vi "GetCalibration.vi"(8 "error in (no error)":errorcluster, 11 "ByteGSWebAPI-V0 in":refnum<class "ByteGSWebAPI-V0.lvclass">) -> (0 "error out":errorcluster, 3 "ByteGSWebAPI-V0 out":refnum<class "ByteGSWebAPI-V0.lvclass">, 4 "body":string, 6 "headers":string)   [LabVIEW 2019, in "ByteGSWebAPI.lvlib" / "ByteGSWebAPI-V0.lvclass"]
uses:
  ByteGSWebAPI-V0.lvclass
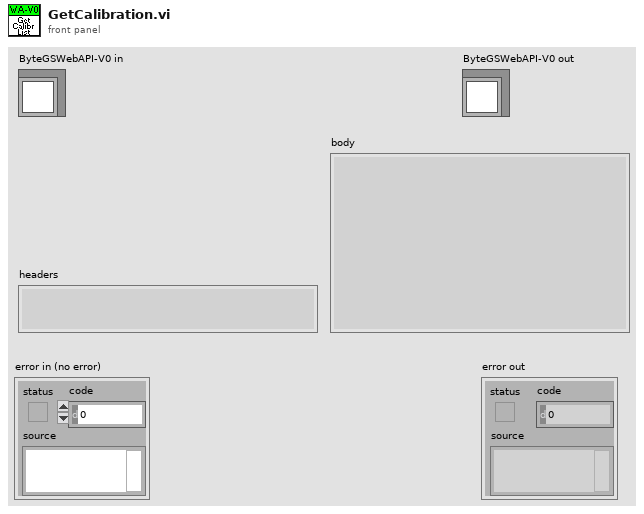
[diagram p1: front panel]
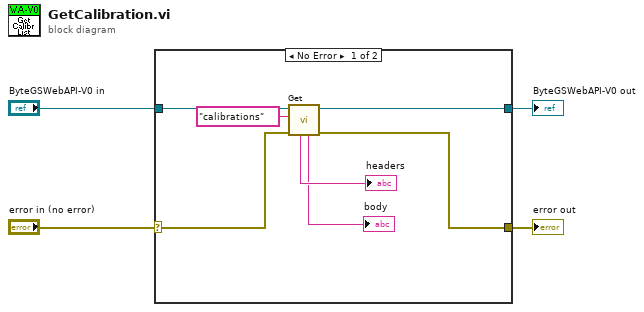
[diagram p0: block diagram]
diagram:
  n1 = case shown="No Error" "error in (no error)" {
    selector: "error in (no error)" -> [w8 w13]
    tunnel: [w5 w13] -> w3
    tunnel: [w10 w12] -> w1
    tunnel: "ByteGSWebAPI-V0 in" -> [w11 w12]
    frame No Error {
      n2 = call-dynamic "Get.vi"("error in (no error)"=w8, "Request"="calibrations" ("Parameter"), "ByteGSWebAPI-V0 in"=w11) -> ("error out"=w5:errorcluster, "ByteGSWebAPI-V0 out"=w10:refnum<class "ByteGSWebAPI-V0.lvclass">, "body"=→"body":string, "headers"=→"headers":string)  [unwired: 5 in]
    }
    frame Error {
    }
  }
  "error out" <- w3
  "ByteGSWebAPI-V0 out" <- w1
